vi "Write.vi"(8 "error in (no error)":errorcluster, 10 "Log Data":T1={"Time"=timestamp(0 s since 1904-01-01), "Level"=enum."INFO", "Logger"="", "Message"="", "Arguments"=[]} {"Time" format="%<%x %.3X>T"}, 11 "Text File - Binary in":refnum<class "Text File - Binary.lvclass">) -> (0 "error out":errorcluster, 3 "Text File - Binary out":refnum<class "Text File - Binary.lvclass">)   [LabVIEW 2019, in "TSC Event Logger.lvlib" / "Text File - Binary.lvclass"]
doc: "Polymorphic, selectable constructor for making a binary event log sink type.\n\n<b>Code Developed By:</b>\nTechnology Service Corporation\nBloomington, IN 47403\nwww.tsc.com/atcs\n\nDeveloper:\nDaniel Coons"
uses:
  Text File - Binary.lvclass
  C:/Development/Open Source/tsc-event-logger/Log Sinks/Log Sinks.lvclass
  C:/Development/Open Source/tsc-event-logger/Log Sinks/Text File/Text File.lvclass
  Log Data.ctl
  Log/Event Level.ctl
  Text File/Text File.lvclass/Text File.ctl
  Text File/Text File.lvclass
  Log Sinks.lvclass
  TSC Event Logger.lvlib
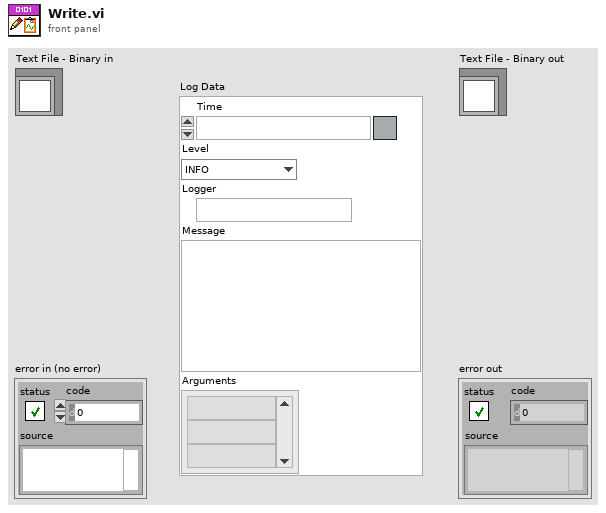
[diagram p1: front panel]
types:
  T1 = typedef "TSC Event Logger.lvlib/Log Data.ctl" = cluster{"Time":timestamp, "Level":T2, "Logger":string, "Message":string, "Arguments":string[]}
  T2 = typedef "TSC Event Logger.lvlib/Event Level.ctl" = enum16{"OFF", "TRACE", "DEBUG", "INFO", "WARN", "ERROR", "FATAL"}
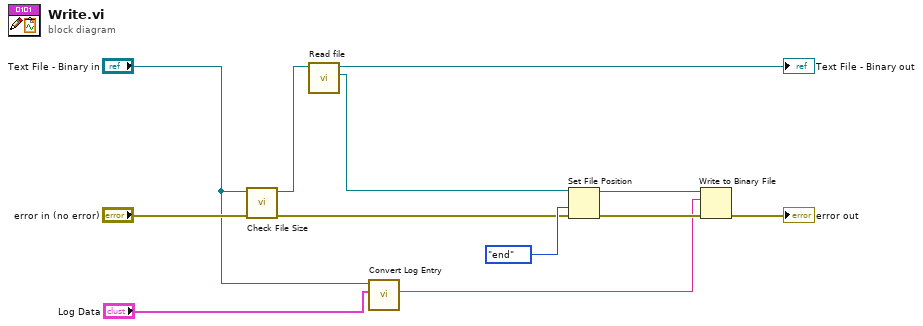
[diagram p0: block diagram]
diagram:
  n1 = call "Check File Size.vi"("error in (no error)"="error in (no error)", "Text File in"="Text File - Binary in") -> ("error out"=w2:errorcluster, "Text File out"=w5:refnum<class "Text File - Binary.lvclass">)  [unwired: 8 in]
  n2 = call "Read file.vi"("Text File in"=w5) -> ("file"=w3:refnum<file>, "Text File out"=→"Text File - Binary out":refnum<class "Text File - Binary.lvclass">)  [unwired: 9 in]
  n3 = call "Convert Log Entry.vi"("Log Data"="Log Data", "Log Sink in"="Text File - Binary in") -> ("Log Entry"=w9:string)  [unwired: 9 in]
  n4 = Set File Position(refnum=w3, from (0:start)=enum16{"start", "end", "current"}."end", error in=w2) -> (refnum out=w10:refnum<file>, error out=w12:errorcluster)  [unwired: 1 in]
  n5 = Write to Binary File(file (use dialog)=w10, data=w9, error in=w12) -> (error out=→"error out":errorcluster)  [unwired: 3 in, 2 out]
